vi "PH_Beckhoff-16BB.PSDBChillerThread.vi"(0 "object ref":refnum<vi>, 5 "error in (no error)":errorcluster) -> (19 "error out":errorcluster)   [LabVIEW 2014, in "PH_Beckhoff-16BB.lvlib"]
doc: "This Template-VI contains a loop to exchange data with the PSDB on request.\n\nLicense Agreement for this software:\n\nCopyright (C)\nGesellschaft für Schwerionenforschung, GSI\nPlanckstr. 1\n64291 Darmstadt\nGermany\n\nContact: H.Brand@gsi.de \n\nThis program is free software; you can redistribute it and/or modify it under the terms of the \nGNU General Public License as published by the Free Software Foundation; either version 2 of \nthe license, or (at your option) any later version.\n\nThis program is distributed in the hope that it will be useful, but WITHOUT ANY WARRANTY; \nwithout even the implied warranty of MERCHANTABILITY or FITNESS FOR A PARTICULAR PURPOSE. See \nthe GNU General License for more details (http://www.gnu.org).\n\nGesellschaft für Schwerionenforschung, GSI\nPlanckstr. 1, 64291 Darmstadt, Germany\nFor all questions and ideas contact: M.Richter@gsi.de, H.Brand@gsi.de or D.Beck@gsi.de.\nLast update: 13-JAN-2005"
uses:
  PH_Beckhoff-16BB.lvlib
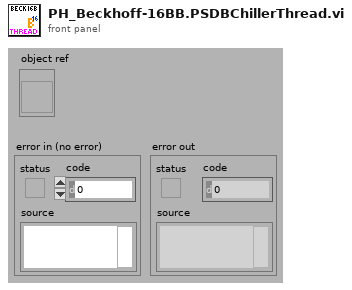
[diagram p1: front panel]
types:
  T1 = typedef "PH_Beckhoff-16BB.lvlib/PH_Beckhoff-16BB.i attribute.ctl" = cluster{"PA Chiller":cluster{"PSDB":cluster{"Status Service ID":i32, "Instance ID":i32, "Data Status":T2, "Ref Status":refnum<vi>, "Error Code":i32}, "Status":cluster{"GUI Ref":refnum<vi>, "Status Service ID":i32, "Status":T3}, "DIs":cluster{"Flow Control":cluster{"GUI Ref":refnum<vi>, "# in Data":i32}, "High-Temp":cluster{"GUI Ref":refnum<vi>, "# in Data":i32}, "Conductivity":cluster{"GUI Ref":refnum<vi>, "# in Data":i32}, "Niveau":cluster{"GUI Ref":refnum<vi>, "# in Data":i32}}, "PSDB Thread":cluster{"Ref":refnum<vi>, "Q-Ref":refnum<queue>}}, "PSDB":cluster{"Shot #":i32, "Subsystem":T4}, "Racktype":string, "PSDB Credentials":T5}
  T2 = typedef "PH_PSDBWriter.lvlib/PH_PSDBWriter.Data Status.ctl" = i16
  T3 = typedef "PH_StatusHandler.lvlib/PH_StatusHandler.Status.ctl" = i16
  T4 = typedef "PH_PSDBWriter.lvlib/PH_PSDBWriter.PHELIX-Subsystems.ctl" = i32
  T5 = typedef "PH_Common.lvlib/PH_Connection.PSDB Credentials.ctl" = cluster{"PW":string, "ID":string, "DS":string}
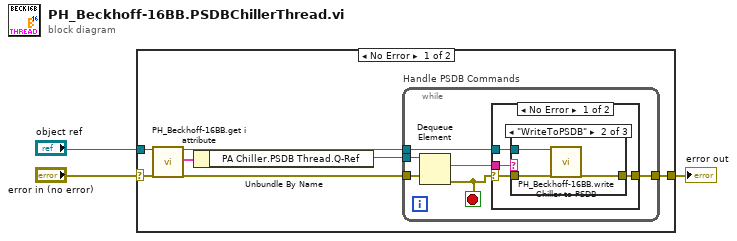
[diagram p0: block diagram]
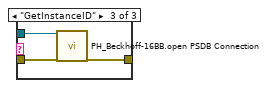
[diagram p3: hidden frame]
diagram:
  n1 = case shown="No Error" "error in (no error)" {
    selector: "error in (no error)" -> [w8 w29]
    tunnel: "object ref" -> [w10 _]
    tunnel: [w4 w29] -> w2
    frame No Error {
      n2 = call "PH_Beckhoff-16BB.get i attribute.vi"("i ref in"=w10, "error in (no error)"=w8) -> ("i ref out"=w9:refnum<vi>, "i attribute"=w6:T1, "error out"=w7:errorcluster)  [unwired: 15 in]
      n3 = Unbundle By Name(w6) -> ("PA Chiller.PSDB Thread.Q-Ref"=w5:refnum<queue>)
      n4 = while "Handle PSDB Commands" {
        tunnel: w9 -> [w16]
        tunnel: w7 -> [w14]
        tunnel: w5 -> [w15]
        tunnel: [w11] -> w4
        stop <- w13 stop-if-true
        n5 = Dequeue Element(queue=w15, error in (no error)=w14) -> (element=w12:string, error out=w13:errorcluster)  [unwired: 1 in, 2 out]
        n6 = case shown="No Error" w13 {
          selector: w13 -> [w19 w28]
          tunnel: w16 -> [w20 _]
          tunnel: w12 -> [w18 _]
          tunnel: [w17 w28] -> w11
          frame No Error {
            n7 = case shown="\"WriteToPSDB\"" w18 {
              tunnel: w20 -> [_ w24 w27]
              tunnel: w19 -> [w21 w23 w26]
              tunnel: [w21 w22 w25] -> w17
              frame Default {
              }
              frame "WriteToPSDB" {
                n8 = call "PH_Beckhoff-16BB.write Chiller to PSDB.vi"("i ref in"=w24, "error IO"=w23) -> ("error out"=w22:errorcluster)  [unwired: 16 in, 1 out]
              }
              frame "GetInstanceID" {
                n9 = call "PH_Beckhoff-16BB.open PSDB Connection.vi"("i ref in"=w27, "error in"=w26) -> ("error out"=w25:errorcluster)  [unwired: 16 in, 1 out]
              }
            }
          }
          frame Error {
          }
        }
      }
    }
    frame Error {
    }
  }
  "error out" <- w2
